vi "Config Store Setting.vi"(0 "VISA resource name":refnum<visa-resource-name>, 7 "Store Config (0:Setting 1)":T1(ring), 11 "error in (no error)":errorcluster) -> (4 "VISA resource name out":refnum<visa-resource-name>, 15 "error out":errorcluster)   [LabVIEW 2010, in "Stanford Research PS300 Series.lvlib"]
doc: "It stores the current configuration setup in the instrument memory."
uses:
  <instrlib>/Stanford Research PS300 Series/Stanford Research PS300 Series.lvlib
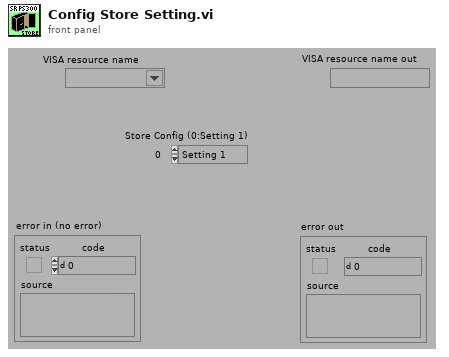
[diagram p1: front panel]
types:
  T1 = enum16{"Setting 1", "Setting 2", "Setting 3", "Setting 4", "Setting 5", "Setting 6", "Setting 7", "Setting 8", "Setting 9"}
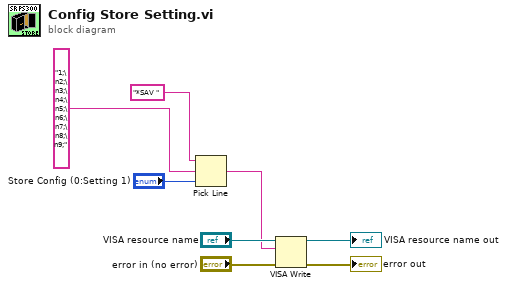
[diagram p0: block diagram]
diagram:
  n1 = Pick Line(string ("")="*SAV ", multi-line string="1;\n2;\n3;\n4;\n5;\n6;\n7;\n8;\n9;", line index="Store Config (0:Setting 1)") -> (output string=w3:string)
  n2 = VISA Write(VISA resource name="VISA resource name", write buffer=w3, error in (no error)="error in (no error)") -> (VISA resource name out=→"VISA resource name out":refnum<visa-resource-name>, error out=→"error out":errorcluster)  [unwired: 1 out]
